vi "Set Server Key File.vi"(10 "Server Key File (.key)":path, 11 "OOP Server in":refnum<class "Servicer.lvclass">) -> (3 "OOP Server out":refnum<class "Servicer.lvclass">)   [LabVIEW 2019, in "gRPC-servicer.lvlib" / "Servicer.lvclass"]
uses:
  Servicer.lvclass
  Servicer.lvclass/Servicer.ctl
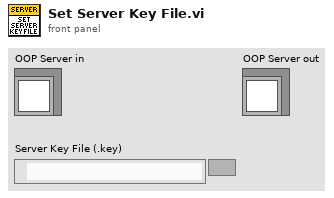
[diagram p1: front panel]
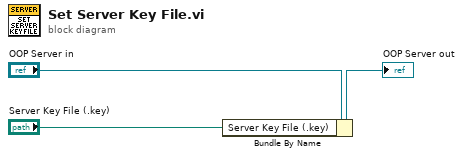
[diagram p0: block diagram]
diagram:
  n1 = Bundle By Name(cluster="OOP Server in", "Server Key File (.key)"="Server Key File (.key)") -> (→"OOP Server out":refnum<class "Servicer.lvclass">)
